vi "Xbox One Controller - Polling Read.vi"() -> ()   [LabVIEW 2011, in "LVH-Xbox-One-Controller.lvlib"]
doc: "This example demonstrates how to read button and axis data from an Xbox One controller using polling."
uses:
  vi.lib/LabVIEW Hacker/Xbox-One-Controller/LVH-Xbox-One-Controller.lvlib
  vi.lib/LabVIEW Hacker/Xbox-One-Controller/Private/Type Defs/Indicators/Controller.ctl
  vi.lib/LabVIEW Hacker/Xbox-One-Controller/Private/Type Defs/Indicators/A.ctl
  vi.lib/LabVIEW Hacker/Xbox-One-Controller/Private/Type Defs/Indicators/B.ctl
  vi.lib/LabVIEW Hacker/Xbox-One-Controller/Private/Type Defs/Indicators/X.ctl
  vi.lib/LabVIEW Hacker/Xbox-One-Controller/Private/Type Defs/Indicators/Y.ctl
  vi.lib/LabVIEW Hacker/Xbox-One-Controller/Private/Type Defs/Indicators/Left Bumper.ctl
  vi.lib/LabVIEW Hacker/Xbox-One-Controller/Private/Type Defs/Indicators/Right Bumper.ctl
  vi.lib/LabVIEW Hacker/Xbox-One-Controller/Private/Type Defs/Indicators/View.ctl
  vi.lib/LabVIEW Hacker/Xbox-One-Controller/Private/Type Defs/Indicators/Menu.ctl
  vi.lib/LabVIEW Hacker/Xbox-One-Controller/Private/Type Defs/Indicators/Thumbstick_Analog.ctl
  vi.lib/LabVIEW Hacker/Xbox-One-Controller/Private/Type Defs/Indicators/Slider.ctl
  vi.lib/LabVIEW Hacker/Xbox-One-Controller/Private/Type Defs/Indicators/DPad.ctl
panel:
  in  "Device Index":i32
  out "Controller":T1={"A Button"=FALSE, "B Button"=FALSE, "X Button"=FALSE, "Y Button"=FALSE, "Left Bumper"=FALSE, "Right Bumper"=FALSE, "View Button"=FALSE, "Menu Button"=FALSE, "Left Stick"={[], []}, "Right Stick"={[], []}, "Trigger"=0, "D-Pad"=5} {"Trigger" scale=32767.0..-32768.0}
  in  "Stop Button":bool
  # "Xbox One Controller  - Polling Read\n\nThis example demonstrates how to read all button and axis data from an Xbox One controller using polling.\n\nInstructions\n1. Select the Device Index associated with the Xbox One Controller.\n     Note: Use the 'Xbox One Controller - Find Controllers' Example in the LabVIEW Example Finder to determine the device index.\n2. Click the Run Arrow.\n3. Notice the controller Icon on the front panel update to match the actual controller state."
  # "Configure"
  # "Controller Data"
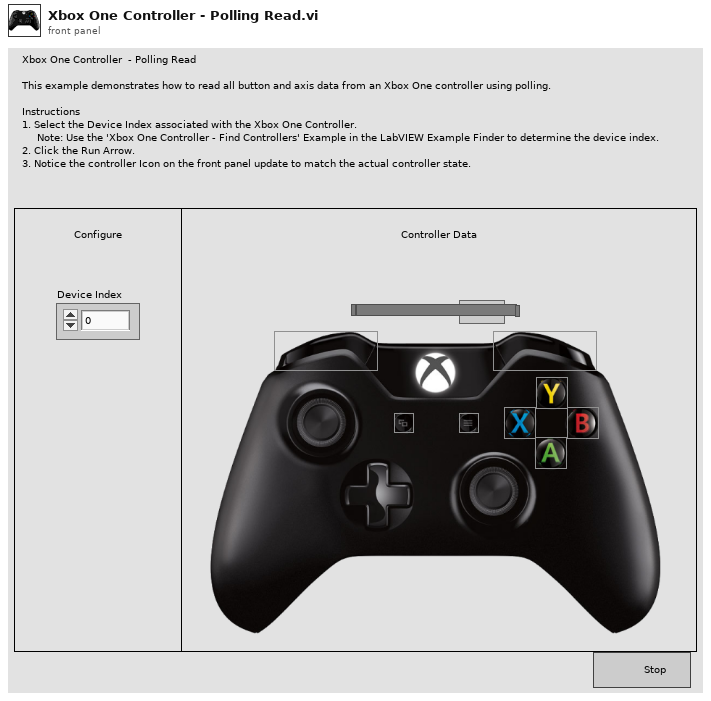
[diagram p1: front panel]
types:
  T1 = typedef "LVH-Xbox-One-Controller.lvlib/Controller.ctl" = cluster{"A Button":T2, "B Button":T3, "X Button":T4, "Y Button":T5, "Left Bumper":T6, "Right Bumper":T7, "View Button":T8, "Menu Button":T9, "Left Stick":T10, "Right Stick":T10, "Trigger":T11, "D-Pad":T12}
  T2 = typedef "LVH-Xbox-One-Controller.lvlib/A.ctl" = bool
  T3 = typedef "LVH-Xbox-One-Controller.lvlib/B.ctl" = bool
  T4 = typedef "LVH-Xbox-One-Controller.lvlib/X.ctl" = bool
  T5 = typedef "LVH-Xbox-One-Controller.lvlib/Y.ctl" = bool
  T6 = typedef "LVH-Xbox-One-Controller.lvlib/Left Bumper.ctl" = bool
  T7 = typedef "LVH-Xbox-One-Controller.lvlib/Right Bumper.ctl" = bool
  T8 = typedef "LVH-Xbox-One-Controller.lvlib/View.ctl" = bool
  T9 = typedef "LVH-Xbox-One-Controller.lvlib/Menu.ctl" = bool
  T10 = typedef "LVH-Xbox-One-Controller.lvlib/Thumbstick_Analog.ctl" = cluster{i32[], i32[]}
  T11 = typedef "LVH-Xbox-One-Controller.lvlib/Slider.ctl" = i32
  T12 = typedef "LVH-Xbox-One-Controller.lvlib/DPad.ctl" = u16
  T13 = typedef "LVH-Xbox-One-Controller.lvlib/Xbox One Controller Ref.ctl" = cluster{"Controller Ref":refnum<k1>, "Event Refnum":refnum<event-registration>, "Worker Ref":refnum<vi>}
  T14 = typedef "LVH-Xbox-One-Controller.lvlib/All Axis Data.ctl" = cluster{"Left Stick":cluster{"X Axis":i32, "Y Axis":i32}, "Right Stick":cluster{"X Axis":i32, "Y Axis":i32}, "Triggers":i32, "D-Pad":T15}
  T15 = typedef "LVH-Xbox-One-Controller.lvlib/DPad Enum.ctl" = enum16{"Idle", "Up", "Up / Right", "Right", "Down / Right", "Down", "Down / Left", "Left", "Up / Left"}
  T16 = typedef "LVH-Xbox-One-Controller.lvlib/All Buttons Visual.ctl" = cluster{"A":T2, "B":T3, "X":T4, "Y":T5, "Left Bumper":T6, "Right Bumper":T7, "View Button":T8, "Menu Button":T9, "Left Stick":T17, "Right Stick":T17}
  T17 = typedef "LVH-Xbox-One-Controller.lvlib/Thumbstick.ctl" = bool
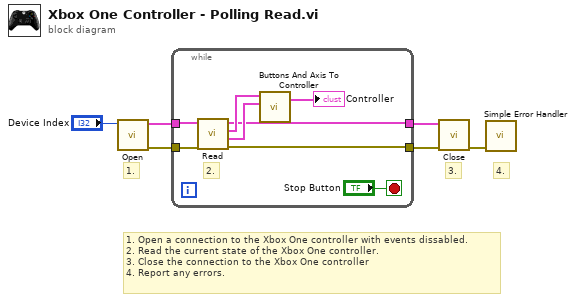
[diagram p0: block diagram]
diagram:
  # "1. Open a connection to the Xbox One controller with events dissabled.\n2. Read the current state of the Xbox One controller.\n3. Close the connection to the Xbox One controller\n4. Report any errors."
  # "4."
  # "3."
  # "1."
  n1 = call "Open.vi"("Device Index"="Device Index") -> ("Error Out"=w5:errorcluster, "Xbox One Controller Ref"=w6:T13)  [unwired: 8 in, 1 out]
  n2 = while {
    tunnel: w5 -> [w13]
    tunnel: w6 -> [w12]
    tunnel: [w9] -> w3
    tunnel: [w8] -> w2
    stop <- "Stop Button" stop-if-true
    # "2."
    n3 = call "Read.vi"("Error In"=w13, "Xbox One Controller Ref"=w12) -> ("Error Out"=w8:errorcluster, "All Axis"=w10:T14, "Buttons"=w11:T16, "Xbox One Controller Ref"=w9:T13)  [unwired: 6 in]
    n4 = call "Buttons And Axis To Controller.vi"("All Axis"=w10, "Buttons"=w11) -> ("Controller"=→"Controller":T1)  [unwired: 5 in]
  }
  n5 = call "Close.vi"("Error In"=w2, "Xbox One Controller Ref"=w3) -> ("Error Out"=w1:errorcluster)  [unwired: 9 in]
  n6 = call <vilib>:"Simple Error Handler.vi"("error in (no error)"=w1) -> ()  [unwired: 4 in, 5 out]
